vi "Auxiliary_Shooter_Motor_Speed_Test.vi"() -> ()   [LabVIEW 2020]
uses:
  <vilib>/Rock Robotics/WPI/ThirdParty/JAS_Junk/TrajLib/LinearFilter_ResetToValue.vi
  <vilib>/Rock Robotics/WPI/ThirdParty/JAS_Junk/TrajLib/LinearFilter_Calculate.vi
  AuxGlobals.vi
  <vilib>/Rock Robotics/WPI/ThirdParty/JAS_Junk/TrajLib/LinearFilter_MovingAverage.vi
  <vilib>/Rock Robotics/WPI/ThirdParty/JAS_Junk/TrajLib/LinearFilter_LowPassBW1.vi
  <vilib>/Rock Robotics/WPI/ThirdParty/JAS_Junk/TrajLib/LinearFilter_LowPassBW2.vi
  <vilib>/Rock Robotics/WPI/ThirdParty/JAS_Junk/TrajLib/LinearFilter_HighPassBW1.vi
  <vilib>/Rock Robotics/WPI/ThirdParty/JAS_Junk/TrajLib/LinearFilter_HighPassBW2.vi
  <vilib>/Rock Robotics/WPI/ThirdParty/JAS_Junk/TrajLib/Trajectory_Library.lvlib
panel:
  out "Avg Motor Out":dbl format="%13.5p"
  out "Avg Speed":dbl format="%13.5p"
  out "Shooter Speed":cluster{"Left Dmd":dbl, "LeftSpeed":dbl}(graph)
  out "Shooter Speed":dbl
  in  "Shooter Dmd":dbl(slide) scale=0.0..5500.0
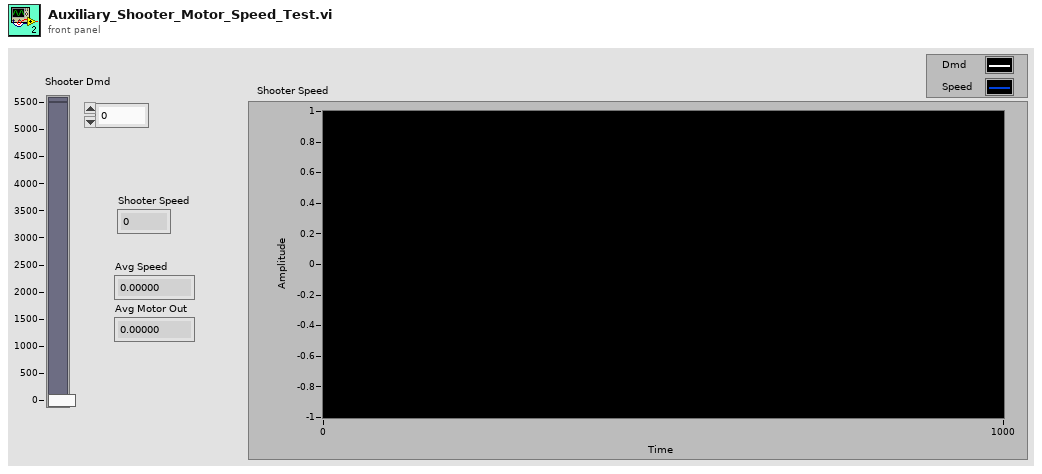
[diagram p1: front panel]
types:
  T1 = typedef "WPI_MotorControlDeviceRef.ctl" = cluster{"DeviceStatus":errorcluster, "Type":T2, "PWM":cluster{"PWM Channel":T3, "DeadBand":T4}, "CAN":cluster{"Device Number":u8, "SetOutput VI Ref":variant, "GetOutput VI Ref":variant, "Enable VI Ref":variant, "Disable VI Ref":variant, "Data":variant}, "Invert":bool, "DIO PWM":cluster{"PWM \"Enable\" Channel":T3, "DIOChannel":T5, "PWM Rate":dbl}}
  T2 = typedef "WPI_MotorControlType.ctl" = enum16{"PWM", "CAN", "DIO PWM"}
  T3 = typedef "FPGA_DIOPWMChannel.ctl" = enum8{"PWM 0", "PWM 1", "PWM 2", "PWM 3", "PWM 4", "PWM 5", "PWM 6", "PWM 7", "PWM 8", "PWM 9", "PWM MXP 0", "PWM MXP 1", "PWM MXP 2", "PWM MXP 3", "PWM MXP 4", "PWM MXP 5", "PWM MXP 6", "PWM MXP 7", "PWM MXP 8", "PWM MXP 9", "Invalid"}
  T4 = typedef "WPI_PWMDeadband.ctl" = cluster{"Name":string, "maxPositivePwm":i32, "minPositivePwm":i32, "centerPwm":i32, "maxNegativePwm":i32, "minNegativePwm":i32, "angularRange":u16}
  T5 = typedef "FPGA_DIOChannel.ctl" = enum8{"DIO 0", "DIO 1", "DIO 2", "DIO 3", "DIO 4", "DIO 5", "DIO 6", "DIO 7", "DIO 8", "DIO 9", "DIO MXP 0", "DIO MXP 1", "DIO MXP 2", "DIO MXP 3", "DIO MXP 4", "DIO MXP 5", "DIO MXP 6", "DIO MXP 7", "DIO MXP 8", "DIO MXP 9", "DIO MXP 10", "DIO MXP 11", "DIO MXP 12", "DIO MXP 13", "DIO MXP 14", "DIO MXP 15", "SPI Port CS1", "SPI Port CS2", "SPI Port CS3", "SPI Port MISO", "SPI Port MOSI", "Invalid"}
  T6 = enum16{"Moving Average", "Low Pass 1st Order Butterworth", "Low Pass 2nd Order Butterworth", "High Pass 1st Order Butterworth", "High Pass 2nd Order Butterworth"}
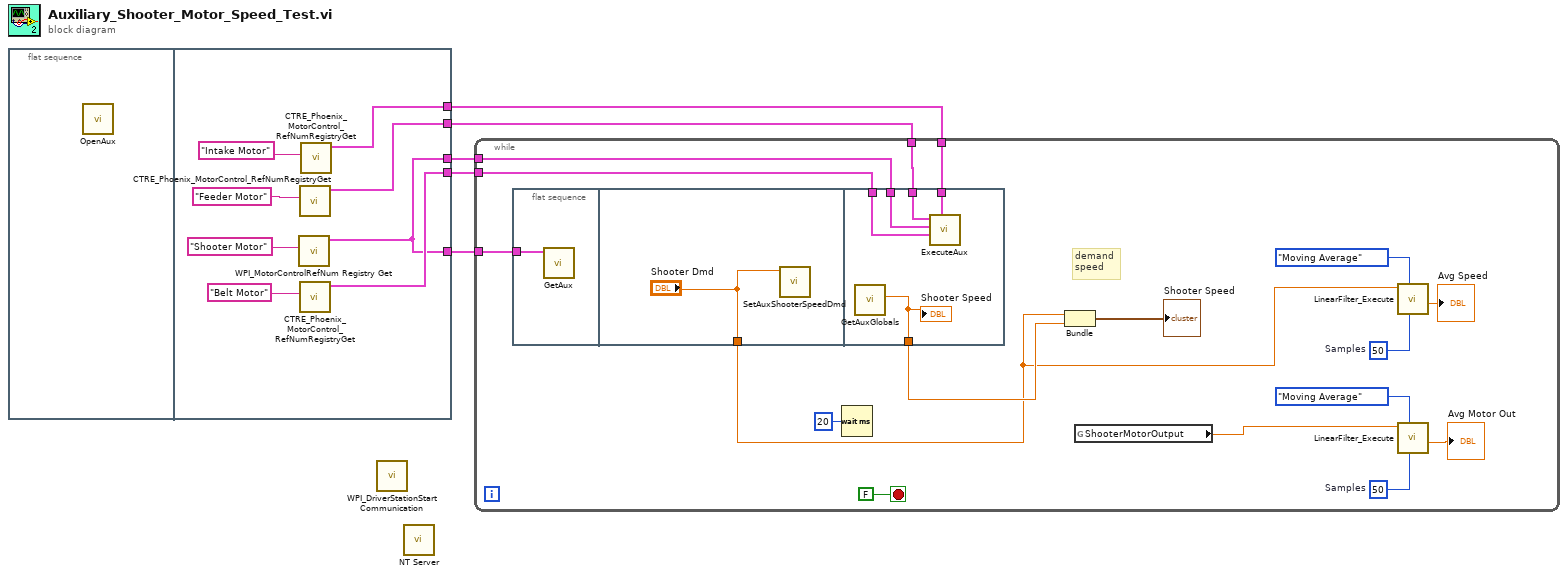
[diagram p0: block diagram]
diagram:
  n1 = flat-sequence {
    tunnel: [w9] -> w5
    tunnel: [w8] -> w4
    tunnel: [w6] -> w3
    tunnel: [w7] -> w2
    tunnel: [w6] -> w1
    frame #0 {
      n2 = call "OpenAux.vi"() -> ()  [unwired: 10 in, 2 out]
    }
    frame #1 {
      n3 = call <vilib>:"WPI_MotorControlRefNum Registry Get.vi"("refnum name"="Shooter Motor") -> ("MotorControlDevRef"=w6:T1)  [unwired: 9 in, 1 out]
      n4 = call <vilib>:"CTRE_Phoenix_MotorControl_RefNumRegistryGet.vi"("refnum name"="Feeder Motor") -> ("PhoenixMotorControlDevRef"=w8:T1)  [unwired: 9 in, 1 out]
      n5 = call <vilib>:"CTRE_Phoenix_MotorControl_RefNumRegistryGet.vi"("refnum name"="Belt Motor") -> ("PhoenixMotorControlDevRef"=w7:T1)  [unwired: 9 in, 1 out]
      n6 = call <vilib>:"CTRE_Phoenix_MotorControl_RefNumRegistryGet.vi"("refnum name"="Intake Motor") -> ("PhoenixMotorControlDevRef"=w9:T1)  [unwired: 9 in, 1 out]
    }
  }
  n7 = call <vilib>:"WPI_DriverStationStart Communication.vi"() -> ()  [unwired: 12 in]
  n8 = call <vilib>:"NT Server.vi"() -> ()  [unwired: 12 in]
  n9 = while {
    tunnel: w5 -> [w18]
    tunnel: w4 -> [w17]
    tunnel: w3 -> [w16]
    tunnel: w2 -> [w15]
    tunnel: w1 -> [w14]
    stop <- FALSE stop-if-true
    w24 = 50  # Samples
    w26 = 50  # Samples
    # "demand\nspeed"
    n10 = flat-sequence {
      tunnel: w14 -> [w31]
      tunnel: ["Shooter Dmd"] -> w21
      tunnel: [w37] -> w28
      tunnel: w18 -> [w36]
      tunnel: w17 -> [w35]
      tunnel: w16 -> [w34]
      tunnel: w15 -> [w33]
      frame #0 {
        n11 = call "GetAux.vi"("Shooter Motor"=w31) -> ()  [unwired: 10 in, 1 out]
      }
      frame #1 {
        n12 = call "SetAuxShooterSpeedDmd.vi"("Shooter Demand"="Shooter Dmd") -> ()  [unwired: 11 in]
      }
      frame #2 {
        n13 = call "GetAuxGlobals.vi"() -> ("ShooterRPM"=w37:dbl)  [unwired: 10 in, 1 out]
        "Shooter Speed" <- w37
        n14 = call "ExecuteAux.vi"("Intake Motor"=w36, "Belt Motor"=w33, "Shooter Motor"=w34, "Feeder Motor"=w35) -> ()  [unwired: 7 in, 1 out]
      }
    }
    n15 = Wait (ms)(milliseconds to wait=u32 20) -> ()  [unwired: 1 out]
    n16 = Bundle("Shooter Dmd"=w21, "ShooterRPM"=w28) -> (→"Shooter Speed":cluster{"Shooter Dmd":dbl, "ShooterRPM":dbl})  [unwired: 1 in]
    n17 = global read "AuxGlobals.vi" "ShooterMotorOutput"() -> (w22:dbl)
    n18 = call <vilib>:"LinearFilter_Execute.vi"("Samples"=w24, "Filter Type"=T6."Moving Average", "Input"=w21) -> ("Output"=→"Avg Speed":dbl)  [unwired: 7 in, 1 out]
    n19 = call <vilib>:"LinearFilter_Execute.vi"("Samples"=w26, "Filter Type"=T6."Moving Average", "Input"=w22) -> ("Output"=→"Avg Motor Out":dbl)  [unwired: 7 in, 1 out]
  }
